vi "Cleanup.vi"(8 "error in (no error)":errorcluster, 11 "Humidity Bricklet in":refnum<class "Humidity Bricklet.lvclass">) -> (0 "error out":errorcluster)   [LabVIEW 2011, in "Tinkerforge.lvlib" / "Humidity Bricklet.lvclass"]
doc: "This VI is the child implementation of \"Cleanup.vi\" and releases all synchronization objects of this child object."
uses:
  Humidity Bricklet.lvclass
  Humidity Bricklet.lvclass/Humidity Bricklet.ctl
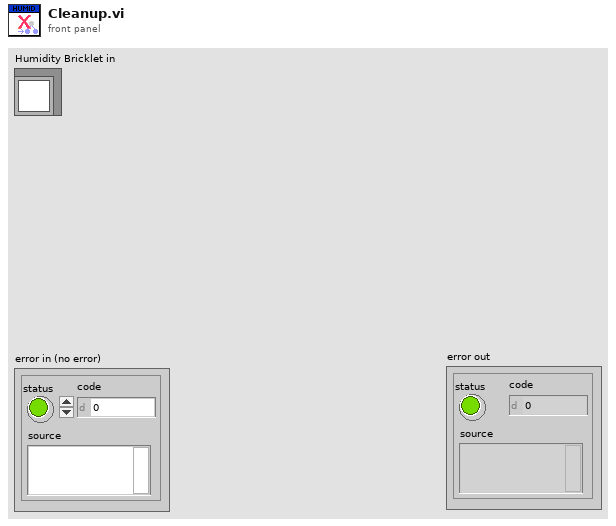
[diagram p1: front panel]
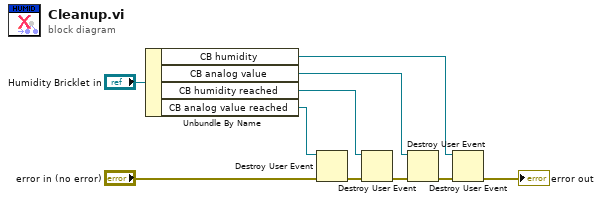
[diagram p0: block diagram]
diagram:
  n1 = Unbundle By Name("Humidity Bricklet in") -> ("CB humidity"=w1:refnum<user-event>, "CB analog value"=w2:refnum<user-event>, "CB humidity reached"=w6:refnum<user-event>, "CB analog value reached"=w8:refnum<user-event>)
  n2 = Destroy User Event(user event=w8, error in="error in (no error)") -> (error out=w7:errorcluster)
  n3 = Destroy User Event(user event=w6, error in=w7) -> (error out=w5:errorcluster)
  n4 = Destroy User Event(user event=w2, error in=w5) -> (error out=w3:errorcluster)
  n5 = Destroy User Event(user event=w1, error in=w3) -> (error out=→"error out":errorcluster)
